vi "Handle Events.vi"(8 "error in (no error)":errorcluster, 11 "MulticolumnListboxEventHandler":refnum<class "MulticolumnListboxEventHandler.lvclass">) -> ()   [LabVIEW 2015, in "ActorEvents.lvlib" / "MulticolumnListboxEventHandler.lvclass"]
uses:
  MulticolumnListboxEventHandler.lvclass
  MulticolumnListboxEventHandler.lvclass/MulticolumnListboxEventHandler.ctl
  IEventHandler/IEventHandler.lvclass/IEventHandler.ctl
  <vilib>/ActorFramework/Message Enqueuer/Message Enqueuer.lvclass/Message Enqueuer.ctl
  IEventAggregator Messages/EventDataMessage/EventDataMessage.lvclass/EventDataMessage.ctl
  IEventAggregator Messages/ControlDragStartingMsg/ControlDragStartingMsg.lvclass/ControlDragStartingMsg.ctl
  IEventAggregator Messages/ControlMouseDownMsg/ControlMouseDownMsg.lvclass/ControlMouseDownMsg.ctl
  IEventAggregator Messages/ControlKeyDownMsg/ControlKeyDownMsg.lvclass/ControlKeyDownMsg.ctl
  IEventAggregator Messages/ListboxEditCellMsg/ListboxEditCellMsg.lvclass/ListboxEditCellMsg.ctl
  <vilib>/event_ctls.llb/lveventtype.ctl
  IEventAggregator Messages/EventDataMessage/Read Discarded.vi
  IEventAggregator Messages/ControlDragStartingMsg/Accessors/Read Data.vi
  IEventAggregator Messages/ControlDragStartingMsg/Accessors/Read Drag Mode.vi
  IEventAggregator Messages/ControlMouseDownMsg/Accessors/Read Button.vi
  IEventAggregator Messages/ControlMouseDownMsg/Accessors/Read Mods.vi
  IEventAggregator Messages/ControlMouseDownMsg/Accessors/Read PlatMods.vi
  IEventAggregator Messages/ControlKeyDownMsg/Accessors/Read Char.vi
  IEventAggregator Messages/ControlKeyDownMsg/Accessors/Read VKey.vi
  IEventAggregator Messages/ControlKeyDownMsg/Accessors/Read Mods.vi
  IEventAggregator Messages/ControlKeyDownMsg/Accessors/Read PlatMods.vi
  IEventAggregator Messages/ControlKeyDownMsg/Accessors/Read FocusObj.vi
  IEventAggregator Messages/ListboxEditCellMsg/Accessors/Read String.vi
  IEventHandler/Accessors/Read Timeout [ms].vi
  IEventHandler/Accessors/Read Event Filter.vi
  IEventHandler/Accessors/Read EventAggregator Enqueuer.vi
  IEventHandler/Accessors/Read Timeout Message.vi
  IEventHandler/Accessors/Read Timeout Message Priority.vi
  <vilib>/ActorFramework/Message Priority Queue/Priority Enqueue.vi
  <vilib>/ActorFramework/Message/Message.lvclass
  <vilib>/ActorFramework/Message Enqueuer/Message Enqueuer.lvclass
  IEventFilter/IEventFilter.lvclass
  IEventAggregator Messages/ValueChangeMsg/ValueChangeMsg.lvclass
  IEventAggregator Messages/ControlMouseDownMsg/ControlMouseDownMsg.lvclass
  IEventAggregator Messages/ControlMouseUpMsg/ControlMouseUpMsg.lvclass
  IEventAggregator Messages/ShortcutMenuSelectionMsg/ShortcutMenuSelectionMsg.lvclass
  IEventAggregator Messages/ShortcutMenuActivationMsg/ShortcutMenuActivationMsg.lvclass
  IEventAggregator Messages/ListboxDoubleClickMsg/ListboxDoubleClickMsg.lvclass
  IEventAggregator Messages/ListboxEditCellMsg/ListboxEditCellMsg.lvclass
  IEventAggregator Messages/ControlMouseEnterMsg/ControlMouseEnterMsg.lvclass
  IEventAggregator Messages/ControlMouseLeaveMsg/ControlMouseLeaveMsg.lvclass
  IEventAggregator Messages/ControlKeyDownMsg/ControlKeyDownMsg.lvclass
  IEventAggregator Messages/ControlKeyUpMsg/ControlKeyUpMsg.lvclass
  IEventAggregator Messages/ControlDropMsg/ControlDropMsg.lvclass
  IEventAggregator Messages/ControlDragStartingMsg/ControlDragStartingMsg.lvclass
  IEventAggregator Messages/ControlDragOverMsg/ControlDragOverMsg.lvclass
  IEventAggregator Messages/ControlDragEndedMsg/ControlDragEndedMsg.lvclass
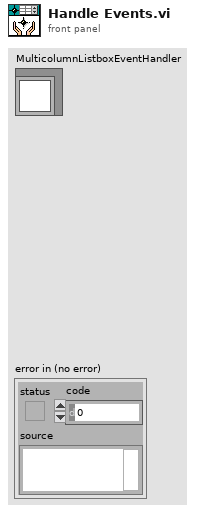
[diagram p1: front panel]
types:
  T1 = typedef "ActorEvents.lvlib/IEventFilter.lvclass/EventFilter Reference.ctl" = refnum<data-value>
  T2 = typedef "Actor Framework.lvlib/Message Enqueuer.lvclass/Message Priority.ctl" = enum16{"Low", "Normal", "High"}
  T3 = typedef "lveventtype.ctl" = enum32{"Null", "Timeout", "Annotation Menu Selection", "Annotation Menu Selection?", "App Instance Close", "App Instance Close?", "Autoscale Range Change", "Bookmark Info Change", "Cell Edit", "Cell Edit?", "Cursor Grab", "Cursor Grab?", "Cursor Menu Selection", "Cursor Menu Selection?", "Cursor Move", "Cursor Release", "Data Change", "Direction Change", "Display State Change", "Drag Ended", "Drag Enter", "Drag Leave", "Drag Over", "Drag Source Update", "Drag Starting", "Drag Starting?", "Drop", "Exec State Change", "Key Down", "Key Down?", "Key Repeat", "Key Repeat?", "Key Up", "Listbox Double Click", "Menu Activation?", "Menu Selection (App)", "Menu Selection? (App)", "Menu Selection (User)", "Mouse Down", "Mouse Down?", "Mouse Enter", "Mouse Leave", "Mouse Move", "Mouse Up", "Mouse Wheel", "NI Security User Change (App)", "Pane Size", "Panel Close", "Panel Close?", "Panel Resize", "Plot Attribute Change", "Scale Range Change", "Shortcut Menu Activation?", "Shortcut Menu Selection (App)", "Shortcut Menu Selection? (App)", "Shortcut Menu Selection (User)", "Tree Double Click", "Tree Drag", "Tree Drag?", "Tree Drop", "Tree Drop?", "Tree Item Close", "Tree Item Close?", "Tree Item Open", "Tree Item Open?", "User Event", "Value Change"}
  T4 = typedef "LVPoint32TypeDef.ctl" = cluster{"Horizontal":i32, "Vertical":i32}
  T5 = cluster{"Shift":bool, "Ctrl":bool, "Alt":bool, "Cmd":bool, "Opt":bool}
  T6 = cluster{"data name":string, "drag data":variant}[]
  T7 = typedef "eventvkey.ctl" = enum16{"ASCII", "Enter", "Return", "Shift", "Ctrl", "Alt", "Cmd", "Opt", "Caps", "NumLock", "Clear", "Break", "Up", "Down", "Left", "Right", "Insert", "Delete", "Home", "End", "PageUp", "PageDown", "Escape", "Help", "Pause", "ScrollLock", "F1", "F2", "F3", "F4", "F5", "F6", "F7", "F8", "F9", "F10", "F11", "F12", "F13", "F14", "F15", "F16", "F17", "F18", "F19", "F20", "F21", "F22", "F23", "F24", "Play", "VolumeUp", "VolumeDown", "Mute", "Two Byte Char"}
  T8 = typedef "LVRowAndColumnTypeDef.ctl" = cluster{"Row":i32, "Column":i32}
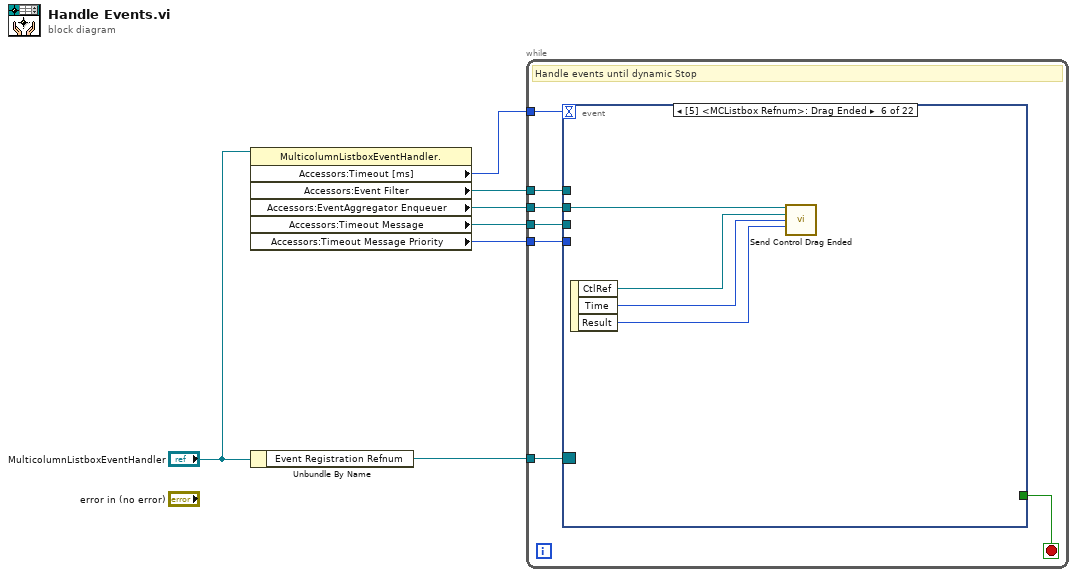
[diagram p0: block diagram]
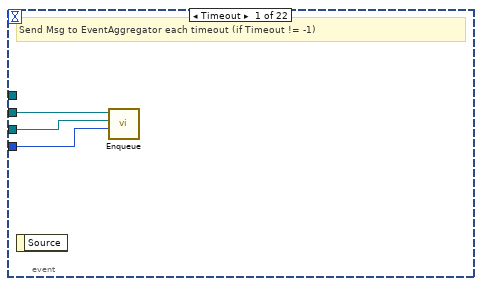
[diagram p2: hidden frame]
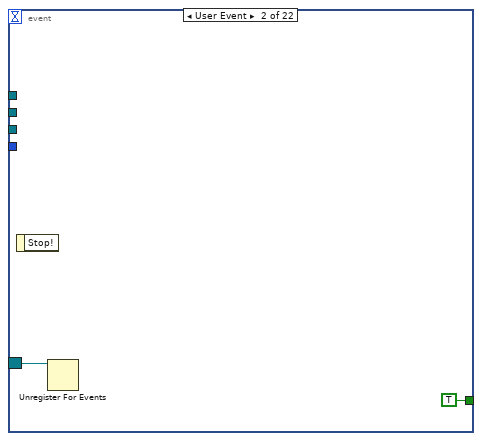
[diagram p3: hidden frame]
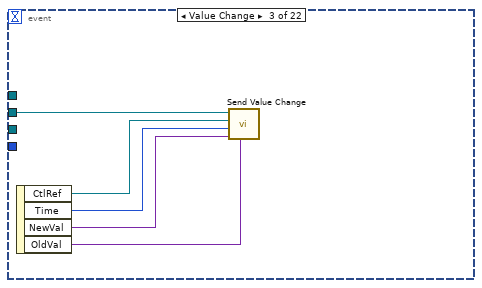
[diagram p4: hidden frame]
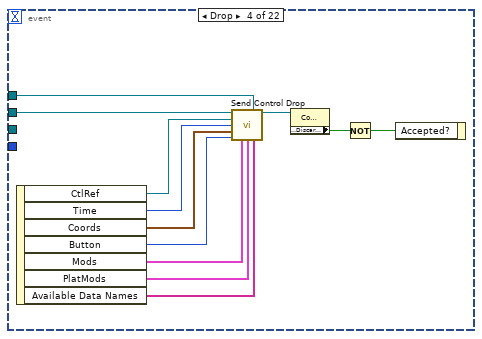
[diagram p5: hidden frame]
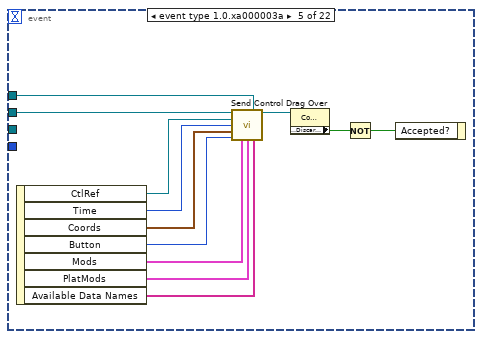
[diagram p6: hidden frame]
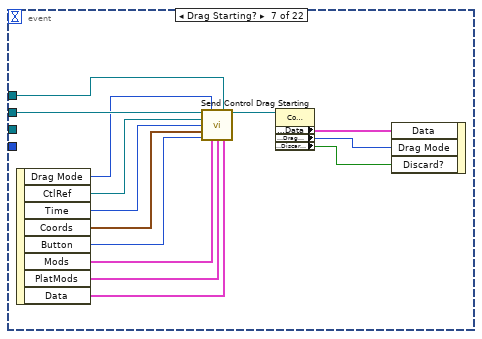
[diagram p7: hidden frame]
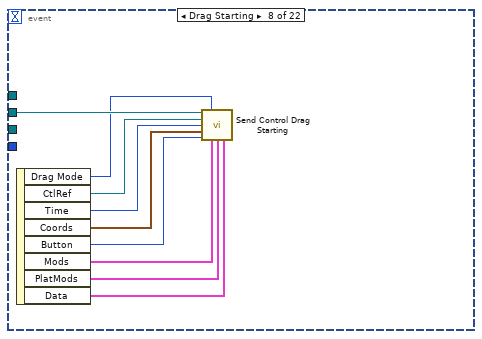
[diagram p8: hidden frame]
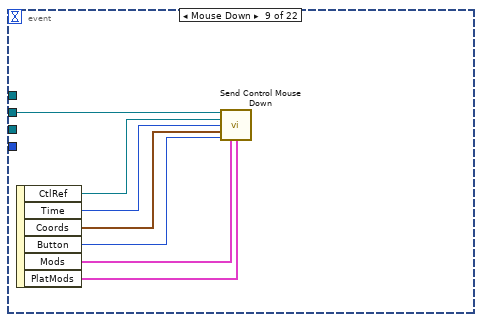
[diagram p9: hidden frame]
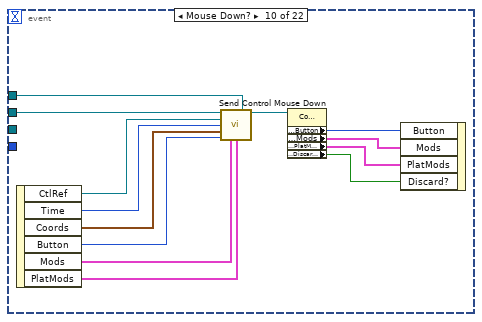
[diagram p10: hidden frame]
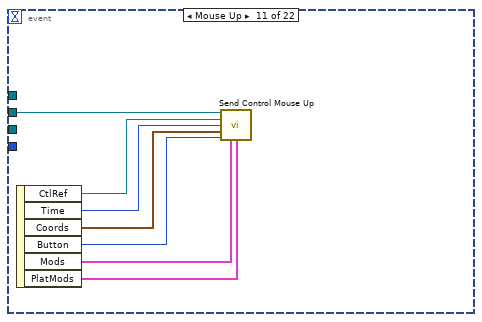
[diagram p11: hidden frame]
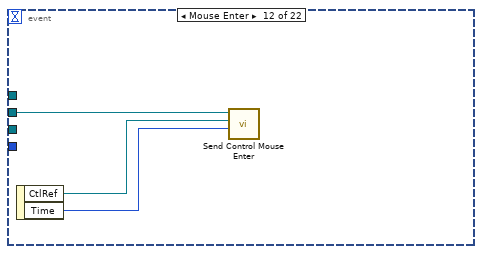
[diagram p12: hidden frame]
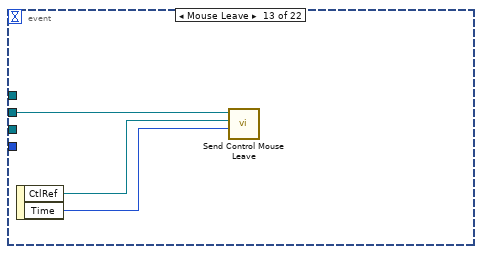
[diagram p13: hidden frame]
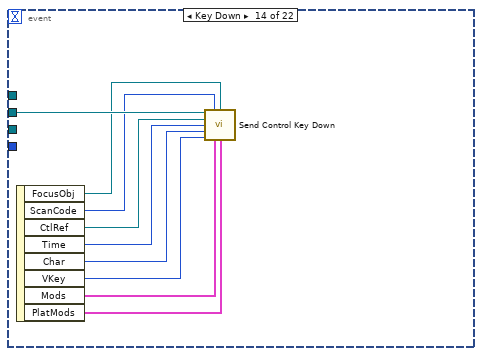
[diagram p14: hidden frame]
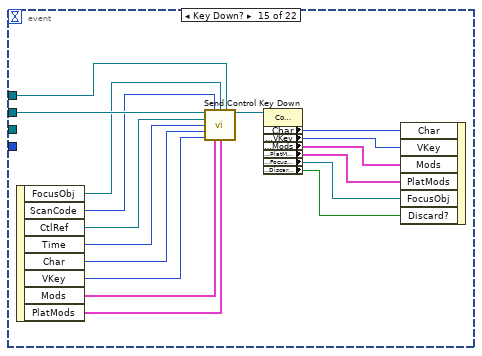
[diagram p15: hidden frame]
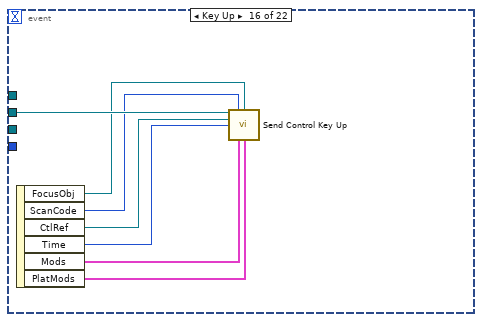
[diagram p16: hidden frame]
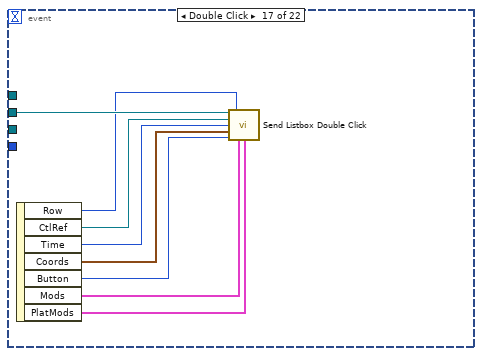
[diagram p17: hidden frame]
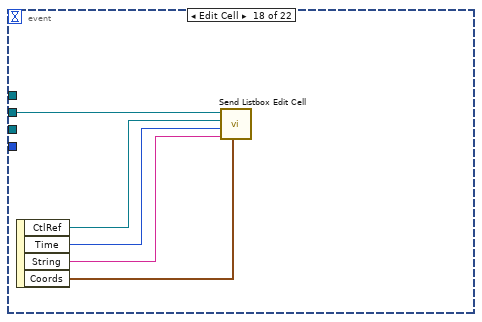
[diagram p18: hidden frame]
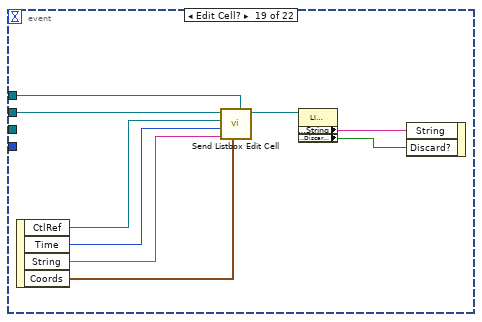
[diagram p19: hidden frame]
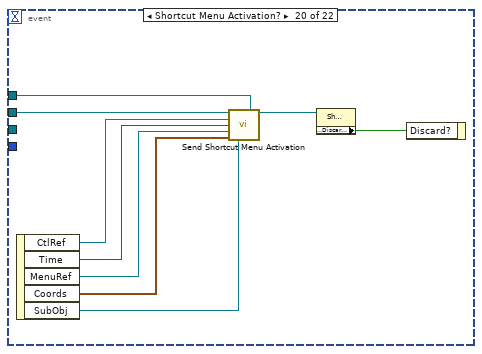
[diagram p20: hidden frame]
diagram:
  n1 = property class="MulticolumnListboxEventHandler."(reference="MulticolumnListboxEventHandler") -> ("Accessors:Timeout [ms]"=w5:i32, "Accessors:Event Filter"=w3:T1, "Accessors:EventAggregator Enqueuer"=w4:refnum<class "Message Enqueuer.lvclass">, "Accessors:Timeout Message"=w2:refnum<class "Message.lvclass">, "Accessors:Timeout Message Priority"=w1:T2)  [unwired: 1 in, 2 out]
  n2 = Unbundle By Name("MulticolumnListboxEventHandler") -> ("Event Registration Refnum"=w7:refnum<event-registration>)
  n3 = while {
    tunnel: w7 -> [w14]
    tunnel: w4 -> [w13]
    tunnel: w2 -> [w12]
    tunnel: w1 -> [w11]
    tunnel: w5 -> [w10]
    tunnel: w3 -> [w8]
    stop <- w9 stop-if-true
    # "Handle events until dynamic Stop"
    n4 = event shown="[5] <MCListbox Refnum>: Drag Ended" {
      selector: w14 -> [_ w19 _ _ _ _ _ _ _ _ _ _ _ _ _ _ _ _ _ _ _ _]
      dyn-events: _ -> [_ _ _ _ _ _ _ _ _ _ _ _ _ _ _ _ _ _ _ _ _ _]
      timeout: w10 -> [_ _ _ _ _ _ _ _ _ _ _ _ _ _ _ _ _ _ _ _ _ _]
      tunnel: [_ TRUE ("Stop!") _ _ _ _ _ _ _ _ _ _ _ _ _ _ _ _ _ _ _ _] -> w9
      tunnel: w13 -> [w17 _ w24 w34 w46 w52 w66 w75 w82 w95 w102 w105 w108 w117 w134 w141 w149 w154 w163 w172 w182 w193]
      tunnel: w12 -> [w16 _ _ _ _ _ _ _ _ _ _ _ _ _ _ _ _ _ _ _ _ _]
      tunnel: w11 -> [w15 _ _ _ _ _ _ _ _ _ _ _ _ _ _ _ _ _ _ _ _ _]
      tunnel: w8 -> [_ _ _ w25 w37 _ w57 _ _ w88 _ _ _ _ w125 _ _ _ w158 w166 _ w186]
      event Timeout {
        # "Send Msg to EventAggregator each timeout (if Timeout != -1)"
        n5 = event-data() -> ()  [unwired: 1 in, 1 out]
        n6 = call <vilib>:"Enqueue.vi"("Message Priority (Normal)"=w15, "Message"=w16, "Message Enqueuer in"=w17) -> ()  [unwired: 7 in, 2 out]
      }
      event User Event {
        n7 = event-data() -> ()  [unwired: 1 in, 1 out]
        n8 = Unregister For Events(event registration refnum=w19) -> ()  [unwired: 1 in, 1 out]
      }
      event Value Change {
        n9 = event-data() -> ("CtlRef"=w21:refnum<vi>, "Time"=w23:u32, "NewVal"=w22:variant, "OldVal"=w20:variant)  [unwired: 1 in]
        n10 = call "Send Value Change.vi"("Old Value"=w20, "New Value"=w22, "Time"=w23, "Ctl Refnum"=w21, "Message Enqueuer in"=w24) -> ()  [unwired: 6 in, 1 out]
      }
      event Drop {
        n11 = event-data() -> ("CtlRef"=w32:refnum<vi>, "Time"=w31:u32, "Coords"=w30:T4, "Button"=w29:u16, "Mods"=w28:cluster{"Double Click":bool, "Menu Key":bool}, "PlatMods"=w27:T5, "Available Data Names"=w26:string[])  [unwired: 1 in]
        n12 = call "Send Control Drop.vi"("Message Enqueuer in"=w34, "EventFilter Reference"=w25, "CtlRef"=w32, "Time"=w31, "Coords"=w30, "Button"=w29, "Mods"=w28, "PlatMods"=w27, "Available Data Names"=w26) -> ("Filtered EventDataMessage"=w36:refnum<class "ControlDropMsg.lvclass">)  [unwired: 5 in, 1 out]
        n13 = property class="ControlDropMsg.lvclass"(reference=w36) -> ("Accessors:Discarded?"=w35:bool)  [unwired: 1 in, 2 out]
        n14 = Not(x=w35) -> (.not. x?=w33:bool)
        n15 = event-data("Accepted?"=w33) -> ()  [unwired: 1 in, 1 out]
      }
      event event type 1.0.xa000003a {
        n16 = event-data() -> ("CtlRef"=w44:refnum<vi>, "Time"=w43:u32, "Coords"=w42:T4, "Button"=w41:u16, "Mods"=w40:cluster{"Double Click":bool, "Menu Key":bool}, "PlatMods"=w39:T5, "Available Data Names"=w38:string[])  [unwired: 1 in]
        n17 = call "Send Control Drag Over.vi"("Message Enqueuer in"=w46, "EventFilter Reference"=w37, "CtlRef"=w44, "Time"=w43, "Coords"=w42, "Button"=w41, "Mods"=w40, "PlatMods"=w39, "Available Data Names"=w38) -> ("ControlDragOverMsg Out"=w48:refnum<class "ControlDragOverMsg.lvclass">)  [unwired: 5 in, 1 out]
        n18 = property class="ControlDragOverMsg.lvclass"(reference=w48) -> ("Accessors:Discarded?"=w47:bool)  [unwired: 1 in, 2 out]
        n19 = Not(x=w47) -> (.not. x?=w45:bool)
        n20 = event-data("Accepted?"=w45) -> ()  [unwired: 1 in, 1 out]
      }
      event Drag Ended {
        n21 = event-data() -> ("CtlRef"=w51:refnum<vi>, "Time"=w50:u32, "Result"=w49:enum16{"Drop Cancel", "Drop Move", "Drop Copy"})  [unwired: 1 in]
        n22 = call "Send Control Drag Ended.vi"("Message Enqueuer in"=w52, "CtlRef"=w51, "Time"=w50, "Result"=w49) -> ()  [unwired: 10 in, 2 out]
      }
      event Drag Starting? {
        n23 = event-data() -> ("Drag Mode"=w58:enum32{"copy or move", "copy only", "move only"}, "CtlRef"=w65:refnum<vi>, "Time"=w64:u32, "Coords"=w63:T4, "Button"=w62:u16, "Mods"=w61:cluster{"Double Click":bool, "Menu Key":bool}, "PlatMods"=w60:T5, "Data"=w59:T6)  [unwired: 1 in]
        n24 = call "Send Control Drag Starting.vi"("Message Enqueuer in"=w66, "Drag Mode"=w58, "EventFilter Reference"=w57, "CtlRef"=w65, "Time"=w64, "Coords"=w63, "Button"=w62, "Mods"=w61, "PlatMods"=w60, "Data"=w59) -> ("Filtered EventDataMessage"=w56:refnum<class "ControlDragStartingMsg.lvclass">)  [unwired: 4 in, 1 out]
        n25 = property class="ControlDragStartingMsg.lvclass"(reference=w56) -> ("Accessors:Data"=w54:T6, "Accessors:Drag Mode"=w53:enum32{"copy or move", "copy only", "move only"}, "Accessors:Discarded?"=w55:bool)  [unwired: 1 in, 2 out]
        n26 = event-data("Data"=w54, "Drag Mode"=w53, "Discard?"=w55) -> ()  [unwired: 1 in, 1 out]
      }
      event Drag Starting {
        n27 = event-data() -> ("Drag Mode"=w67:enum32{"copy or move", "copy only", "move only"}, "CtlRef"=w74:refnum<vi>, "Time"=w73:u32, "Coords"=w72:T4, "Button"=w71:u16, "Mods"=w70:cluster{"Double Click":bool, "Menu Key":bool}, "PlatMods"=w69:T5, "Data"=w68:T6)  [unwired: 1 in]
        n28 = call "Send Control Drag Starting.vi"("Message Enqueuer in"=w75, "Drag Mode"=w67, "CtlRef"=w74, "Time"=w73, "Coords"=w72, "Button"=w71, "Mods"=w70, "PlatMods"=w69, "Data"=w68) -> ()  [unwired: 5 in, 2 out]
      }
      event Mouse Down {
        n29 = event-data() -> ("CtlRef"=w81:refnum<vi>, "Time"=w80:u32, "Coords"=w79:T4, "Button"=w78:u16, "Mods"=w77:cluster{"Double Click":bool, "Menu Key":bool}, "PlatMods"=w76:T5)  [unwired: 1 in]
        n30 = call "Send Control Mouse Down.vi"("Message Enqueuer in"=w82, "Ctl Refnum"=w81, "Time"=w80, "Coords"=w79, "Button"=w78, "Mods"=w77, "PlatMods"=w76) -> ()  [unwired: 7 in, 2 out]
      }
      event Mouse Down? {
        n31 = event-data() -> ("CtlRef"=w94:refnum<vi>, "Time"=w93:u32, "Coords"=w92:T4, "Button"=w91:u16, "Mods"=w90:cluster{"Double Click":bool, "Menu Key":bool}, "PlatMods"=w89:T5)  [unwired: 1 in]
        n32 = call "Send Control Mouse Down.vi"("Message Enqueuer in"=w95, "EventFilter Reference"=w88, "Ctl Refnum"=w94, "Time"=w93, "Coords"=w92, "Button"=w91, "Mods"=w90, "PlatMods"=w89) -> ("Filtered EventDataMessage"=w87:refnum<class "ControlMouseDownMsg.lvclass">)  [unwired: 6 in, 1 out]
        n33 = property class="ControlMouseDownMsg.lvclass"(reference=w87) -> ("Accessors:Button"=w86:u16, "Accessors:Mods"=w85:cluster{"Double Click":bool, "Menu Key":bool}, "Accessors:PlatMods"=w84:T5, "Accessors:Discarded?"=w83:bool)  [unwired: 1 in, 2 out]
        n34 = event-data("Button"=w86, "Mods"=w85, "PlatMods"=w84, "Discard?"=w83) -> ()  [unwired: 1 in, 1 out]
      }
      event Mouse Up {
        n35 = event-data() -> ("CtlRef"=w101:refnum<vi>, "Time"=w100:u32, "Coords"=w99:T4, "Button"=w98:u16, "Mods"=w97:cluster{"Double Click":bool, "Menu Key":bool}, "PlatMods"=w96:T5)  [unwired: 1 in]
        n36 = call "Send Control Mouse Up.vi"("Message Enqueuer in"=w102, "Ctl Refnum"=w101, "Time"=w100, "Coords"=w99, "Button"=w98, "Mods"=w97, "PlatMods"=w96) -> ()  [unwired: 8 in, 1 out]
      }
      event Mouse Enter {
        n37 = event-data() -> ("CtlRef"=w104:refnum<vi>, "Time"=w103:u32)  [unwired: 1 in]
        n38 = call "Send Control Mouse Enter.vi"("Time"=w103, "Ctl Refnum"=w104, "Message Enqueuer in"=w105) -> ()  [unwired: 8 in, 1 out]
      }
      event Mouse Leave {
        n39 = event-data() -> ("CtlRef"=w107:refnum<vi>, "Time"=w106:u32)  [unwired: 1 in]
        n40 = call "Send Control Mouse Leave.vi"("Time"=w106, "Ctl Refnum"=w107, "Message Enqueuer in"=w108) -> ()  [unwired: 8 in, 1 out]
      }
      event Key Down {
        n41 = event-data() -> ("FocusObj"=w116:refnum<vi>, "ScanCode"=w115:i16, "CtlRef"=w114:refnum<vi>, "Time"=w113:u32, "Char"=w112:i16, "VKey"=w111:T7, "Mods"=w110:cluster{"Num Pad":bool, "Menu Key":bool}, "PlatMods"=w109:T5)  [unwired: 1 in]
        n42 = call "Send Control Key Down.vi"("Message Enqueuer in"=w117, "ScanCode"=w115, "FocusObj"=w116, "CtlRef"=w114, "Time"=w113, "Char"=w112, "VKey"=w111, "Mods"=w110, "PlatMods"=w109) -> ()  [unwired: 5 in, 2 out]
      }
      event Key Down? {
        n43 = event-data() -> ("FocusObj"=w133:refnum<vi>, "ScanCode"=w132:i16, "CtlRef"=w131:refnum<vi>, "Time"=w130:u32, "Char"=w129:i16, "VKey"=w128:T7, "Mods"=w127:cluster{"Num Pad":bool, "Menu Key":bool}, "PlatMods"=w126:T5)  [unwired: 1 in]
        n44 = call "Send Control Key Down.vi"("Message Enqueuer in"=w134, "ScanCode"=w132, "FocusObj"=w133, "EventFilter Reference"=w125, "CtlRef"=w131, "Time"=w130, "Char"=w129, "VKey"=w128, "Mods"=w127, "PlatMods"=w126) -> ("Filtered EventDataMessage"=w124:refnum<class "ControlKeyDownMsg.lvclass">)  [unwired: 4 in, 1 out]
        n45 = property class="ControlKeyDownMsg.lvclass"(reference=w124) -> ("Accessors:Char"=w123:i16, "Accessors:VKey"=w122:T7, "Accessors:Mods"=w121:cluster{"Double Click":bool, "Menu Key":bool}, "Accessors:PlatMods"=w120:T5, "Accessors:FocusObj"=w119:refnum<vi>, "Accessors:Discarded?"=w118:bool)  [unwired: 1 in, 2 out]
        n46 = event-data("Char"=w123, "VKey"=w122, "Mods"=w121, "PlatMods"=w120, "FocusObj"=w119, "Discard?"=w118) -> ()  [unwired: 1 in, 1 out]
      }
      event Key Up {
        n47 = event-data() -> ("FocusObj"=w140:refnum<vi>, "ScanCode"=w139:i16, "CtlRef"=w138:refnum<vi>, "Time"=w137:u32, "Mods"=w136:cluster{"Num Pad":bool, "Menu Key":bool}, "PlatMods"=w135:T5)  [unwired: 1 in]
        n48 = call "Send Control Key Up.vi"("Message Enqueuer in"=w141, "ScanCode"=w139, "FocusObj"=w140, "Ctl Refnum"=w138, "Time"=w137, "Mods"=w136, "PlatMods"=w135) -> ()  [unwired: 8 in, 1 out]
      }
      event Double Click {
        n49 = event-data() -> ("Row"=w142:i32, "CtlRef"=w148:refnum<vi>, "Time"=w147:u32, "Coords"=w146:T4, "Button"=w145:u16, "Mods"=w144:cluster{"Double Click":bool, "Menu Key":bool}, "PlatMods"=w143:T5)  [unwired: 1 in]
        n50 = call "Send Listbox Double Click.vi"("Message Enqueuer in"=w149, "Row"=w142, "Ctl Refnum"=w148, "Time"=w147, "Coords"=w146, "Button"=w145, "Mods"=w144, "PlatMods"=w143) -> ()  [unwired: 7 in, 1 out]
      }
      event Edit Cell {
        n51 = event-data() -> ("CtlRef"=w153:refnum<vi>, "Time"=w152:u32, "String"=w151:string, "Coords"=w150:T8)  [unwired: 1 in]
        n52 = call "Send Listbox Edit Cell.vi"("Coords"=w150, "String"=w151, "Time"=w152, "CtlRef"=w153, "Message Enqueuer in"=w154) -> ()  [unwired: 5 in, 2 out]
      }
      event Edit Cell? {
        n53 = event-data() -> ("CtlRef"=w162:refnum<vi>, "Time"=w161:u32, "String"=w160:string, "Coords"=w159:T8)  [unwired: 1 in]
        n54 = call "Send Listbox Edit Cell.vi"("EventFilter Reference"=w158, "Coords"=w159, "String"=w160, "Time"=w161, "CtlRef"=w162, "Message Enqueuer in"=w163) -> ("Filtered EventDataMessage"=w157:refnum<class "ListboxEditCellMsg.lvclass">)  [unwired: 4 in, 1 out]
        n55 = property class="ListboxEditCellMsg.lvclass"(reference=w157) -> ("Accessors:String"=w156:string, "Accessors:Discarded?"=w155:bool)  [unwired: 1 in, 2 out]
        n56 = event-data("String"=w156, "Discard?"=w155) -> ()  [unwired: 1 in, 1 out]
      }
      event Shortcut Menu Activation? {
        n57 = event-data() -> ("CtlRef"=w167:refnum<vi>, "Time"=w171:u32, "MenuRef"=w168:refnum<k9>, "Coords"=w170:T4, "SubObj"=w169:refnum<vi>)  [unwired: 1 in]
        n58 = call "Send Shortcut Menu Activation.vi"("Message Enqueuer in"=w172, "EventFilter Reference"=w166, "CtlRef"=w167, "Time"=w171, "MenuRef"=w168, "Coords"=w170, "SubObj"=w169) -> ("Filtered EventDataMessage"=w165:refnum<class "ShortcutMenuActivationMsg.lvclass">)  [unwired: 7 in, 1 out]
        n59 = property class="ShortcutMenuActivationMsg.lvcla"(reference=w165) -> ("Accessors:Discarded?"=w164:bool)  [unwired: 1 in, 2 out]
        n60 = event-data("Discard?"=w164) -> ()  [unwired: 1 in, 1 out]
      }
      event Shortcut Menu Selection (User); Shortcut Menu Selection (App) {
        n61 = event-data() -> ("Type"=w175:T3, "CtlRef"=w181:refnum<vi>, "Time"=w180:u32, "ItemTag"=w179:string, "ItemPath"=w178:string, "Coords"=w177:T4, "SubObj"=w176:refnum<vi>)  [unwired: 1 in]
        n62 = Equal?(x=lveventtype."Shortcut Menu Selection (App)", y=w175) -> (x = y?=w174:bool)
        n63 = call "Send Shortcut Menu Selection.vi"("Message Enqueuer in"=w182, "App Item?"=w174, "CtlRef"=w181, "Time"=w180, "Item Tag"=w179, "Item Path"=w178, "Coords"=w177, "SubObj"=w176) -> ()  [unwired: 6 in, 2 out]
      }
      event Shortcut Menu Selection? (App) {
        w185 = TRUE  # App Item?
        n64 = event-data() -> ("CtlRef"=w192:refnum<vi>, "Time"=w191:u32, "ItemTag"=w190:string, "ItemPath"=w189:string, "Coords"=w188:T4, "SubObj"=w187:refnum<vi>)  [unwired: 1 in, 1 out]
        n65 = call "Send Shortcut Menu Selection.vi"("Message Enqueuer in"=w193, "App Item?"=w185, "EventFilter Reference"=w186, "CtlRef"=w192, "Time"=w191, "Item Tag"=w190, "Item Path"=w189, "Coords"=w188, "SubObj"=w187) -> ("Filtered EventDataMessage"=w184:refnum<class "ShortcutMenuSelectionMsg.lvclass">)  [unwired: 5 in, 1 out]
        n66 = property class="ShortcutMenuSelectionMsg.lvclas"(reference=w184) -> ("Accessors:Discarded?"=w183:bool)  [unwired: 1 in, 2 out]
        n67 = event-data("Discard?"=w183) -> ()  [unwired: 1 in, 1 out]
      }
    }
  }
